vi "GetI2C.vi"(8 "error in (no error)":errorcluster, 11 "GrovePi in":refnum<class "GrovePi.lvclass">) -> (0 "error out":errorcluster, 2 "I2C":refnum<class "I2C.lvclass">, 3 "GrovePi out":refnum<class "GrovePi.lvclass">)   [LabVIEW 2014, in "GrovePi.lvclass"]
doc: "Gets the I2C bus used for communications to the GrovePi."
uses:
  GrovePi.lvclass
  I2C/I2C.lvclass
  GrovePi.lvclass/GrovePi.ctl
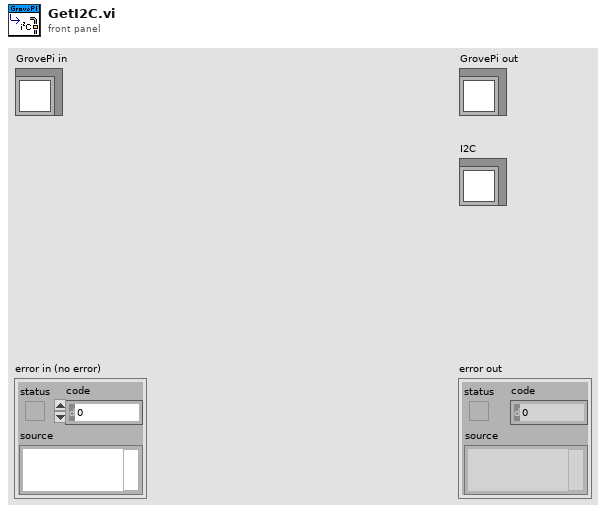
[diagram p1: front panel]
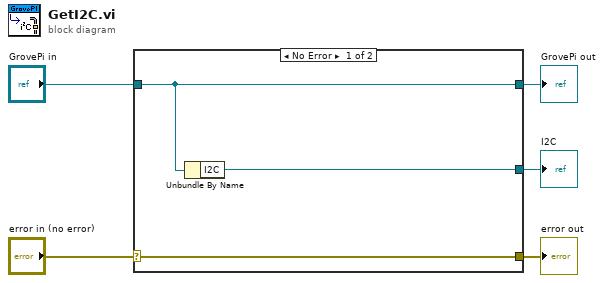
[diagram p0: block diagram]
diagram:
  n1 = case shown="No Error" "error in (no error)" {
    selector: "error in (no error)" -> [w8 w9]
    tunnel: [w8 w9] -> w4
    tunnel: [w7 w10] -> w2
    tunnel: "GrovePi in" -> [w7 w10]
    tunnel: [w6 _] -> w1
    frame No Error {
      n2 = Unbundle By Name(w7) -> ("I2C"=w6:refnum<class "I2C.lvclass">)
    }
    frame Error {
    }
  }
  "error out" <- w4
  "GrovePi out" <- w2
  "I2C" <- w1
